vi "FlatToRichnixnet_grpc_WriteStateRequest.vi"(5 "OutputClusterType":T1, 11 "InputCluster":T4) -> (3 "OutputCluster":T1)   [LabVIEW 2025, in "xnet-grpc_client.lvlib"]
uses:
  nixnet_grpc_WriteStateRequest_Flat.ctl
  nidevice_grpc_Session_Flat.ctl
  nixnet_grpc_WriteState.ctl
  nixnet_grpc_WriteStateValue_Flat.ctl
  nixnet_grpc_LinDiagnosticScheduleChangeRequest_Flat.ctl
  nixnet_grpc_LinDiagnosticSchedule.ctl
  nixnet_grpc_WriteStateRequest.ctl
  nixnet_grpc_WriteStateRequest_state_id_enum/nixnet_grpc_WriteStateRequest_state_id_enum.lvclass
  nixnet_grpc_WriteStateValue_value/nixnet_grpc_WriteStateValue_value.lvclass
  nidevice_grpc_Session.ctl
  nixnet_grpc_WriteStateValue.ctl
  xnet-grpc_client.lvlib
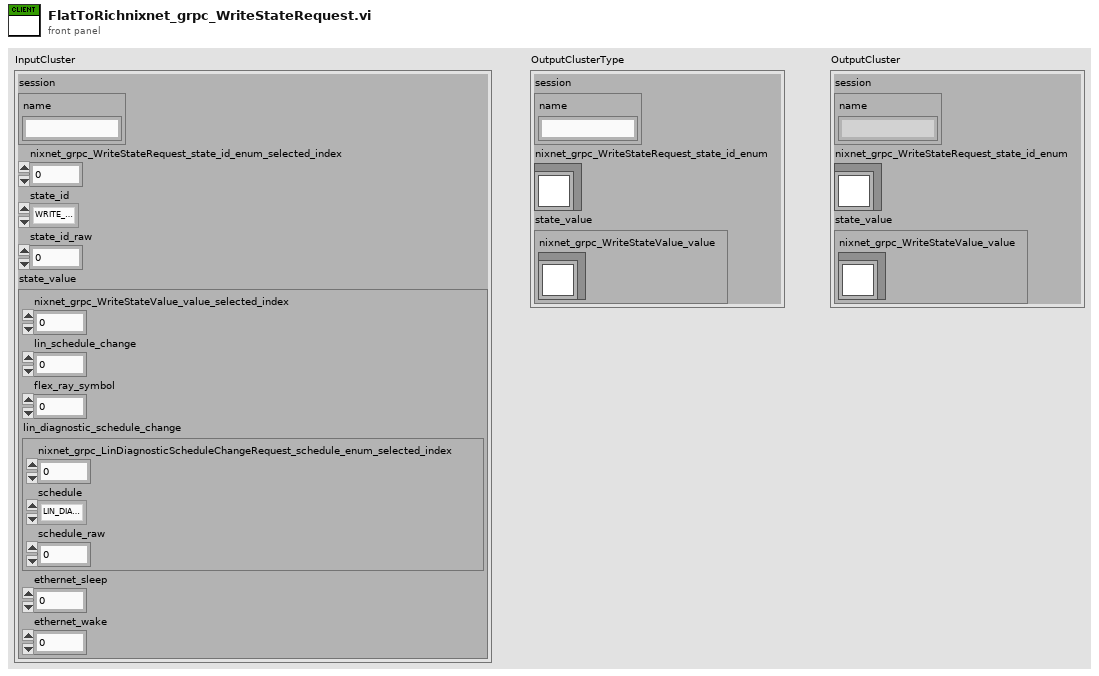
[diagram p1: front panel]
types:
  T1 = typedef "xnet-grpc_client.lvlib/nixnet_grpc_WriteStateRequest.ctl" = cluster{"session":T2, "nixnet_grpc_WriteStateRequest_state_id_enum":refnum<class "nixnet_grpc_WriteStateRequest_state_id_enum.lvclass">, "state_value":T3}
  T2 = typedef "xnet-grpc_client.lvlib/nidevice_grpc_Session.ctl" = cluster{"name":string}
  T3 = typedef "xnet-grpc_client.lvlib/nixnet_grpc_WriteStateValue.ctl" = cluster{"nixnet_grpc_WriteStateValue_value":refnum<class "nixnet_grpc_WriteStateValue_value.lvclass">}
  T4 = typedef "xnet-grpc_client.lvlib/nixnet_grpc_WriteStateRequest_Flat.ctl" = cluster{"session":T5, "nixnet_grpc_WriteStateRequest_state_id_enum_selected_index":i32, "state_id":T6, "state_id_raw":u32, "state_value":T7}
  T5 = typedef "xnet-grpc_client.lvlib/nidevice_grpc_Session_Flat.ctl" = cluster{"name":string}
  T6 = typedef "xnet-grpc_client.lvlib/nixnet_grpc_WriteState.ctl" = enum32{"WRITE_STATE_UNSPECIFIED", "WRITE_STATE_LIN_SCHEDULE_CHANGE", "WRITE_STATE_LIN_DIAGNOSTIC_SCHEDULE_CHANGE", "WRITE_STATE_FLEX_RAY_SYMBOL", "WRITE_STATE_ETHERNET_SLEEP", "WRITE_STATE_ETHERNET_WAKE"}
  T7 = typedef "xnet-grpc_client.lvlib/nixnet_grpc_WriteStateValue_Flat.ctl" = cluster{"nixnet_grpc_WriteStateValue_value_selected_index":i32, "lin_schedule_change":u32, "flex_ray_symbol":u32, "lin_diagnostic_schedule_change":T8, "ethernet_sleep":u32, "ethernet_wake":u32}
  T8 = typedef "xnet-grpc_client.lvlib/nixnet_grpc_LinDiagnosticScheduleChangeRequest_Flat.ctl" = cluster{"nixnet_grpc_LinDiagnosticScheduleChangeRequest_schedule_enum_selected_index":i32, "schedule":T9, "schedule_raw":u32}
  T9 = typedef "xnet-grpc_client.lvlib/nixnet_grpc_LinDiagnosticSchedule.ctl" = enum32{"LIN_DIAGNOSTIC_SCHEDULE_NULL", "LIN_DIAGNOSTIC_SCHEDULE_MASTER_REQ", "LIN_DIAGNOSTIC_SCHEDULE_SLAVE_RESP"}
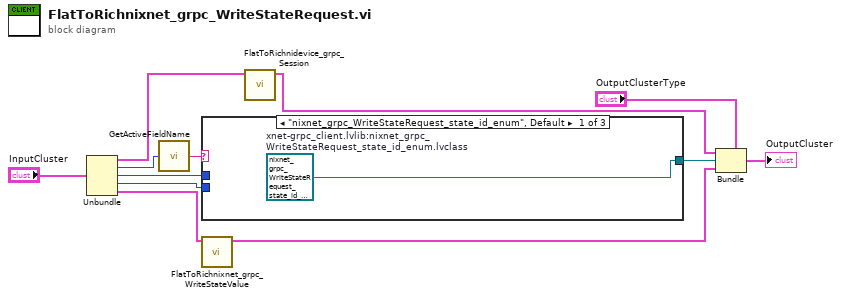
[diagram p0: block diagram]
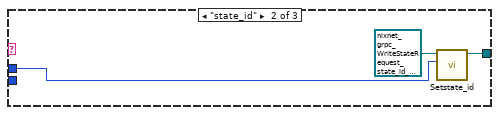
[diagram p2: hidden frame]
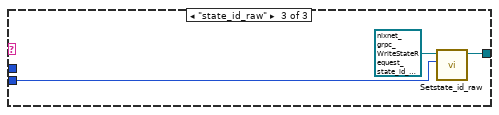
[diagram p3: hidden frame]
diagram:
  n1 = Unbundle "Unbundle"("InputCluster") -> ("session"=w9:T5, "nixnet_grpc_WriteStateRequest_state_id_enum_selected_index"=w7:i32, "state_id"=w4:T6, "state_id_raw"=w3:u32, "state_value"=w2:T7)
  n2 = call "GetActiveFieldName.vi"("protobuf index"=w7) -> ("oneof field name"=w6:string)
  n3 = case "nixnet_grpc_WriteStateRequest_state_id_enum" shown="\"nixnet_grpc_WriteStateRequest_state_id_enum\", Default" w6 {
    tunnel: [w13 w15 w18] -> w5
    tunnel: w4 -> [_ w16 _]
    tunnel: w3 -> [_ _ w19]
    frame "nixnet_grpc_WriteStateRequest_state_id_enum", Default {
      w13 = refnum<class "nixnet_grpc_WriteStateRequest_state_id_enum.lvclass"> refnum  # xnet-grpc_client.lvlib:nixnet_grpc_WriteStateRequest_state_id_enum.lvclass
    }
    frame "state_id" {
      n4 = call "Setstate_id.vi"("Set_Val"=w16, "OneOfTemplate in"=refnum<class "nixnet_grpc_WriteStateRequest_state_id_enum.lvclass"> refnum) -> ("OneOfTemplate out"=w15:refnum<class "nixnet_grpc_WriteStateRequest_state_id_enum.lvclass">)  [unwired: 8 in, 1 out]
    }
    frame "state_id_raw" {
      n5 = call "Setstate_id_raw.vi"("Set_Val"=w19, "OneOfTemplate in"=refnum<class "nixnet_grpc_WriteStateRequest_state_id_enum.lvclass"> refnum) -> ("OneOfTemplate out"=w18:refnum<class "nixnet_grpc_WriteStateRequest_state_id_enum.lvclass">)  [unwired: 8 in, 1 out]
    }
  }
  n6 = call "FlatToRichnixnet_grpc_WriteStateValue.vi"("InputCluster"=w2) -> ("OutputCluster"=w1:T3)  [unwired: 10 in]
  n7 = call "FlatToRichnidevice_grpc_Session.vi"("InputCluster"=w9) -> ("OutputCluster"=w8:T2)  [unwired: 10 in]
  n8 = Bundle "Bundle"(cluster="OutputClusterType", "session"=w8, "nixnet_grpc_WriteStateRequest_state_id_enum"=w5, "state_value"=w1) -> (→"OutputCluster":T1)
